vi "Graph Scale Properties.vi"(1 "Long term plot":refnum<vi>, 3 "Selected Variables":string[][](array[string]), 4 "Legend Rows":i32=5, 5 "error in (no error)":errorcluster, 6 "Short term graph":refnum<vi>) -> (19 "error out":errorcluster)   [LabVIEW 2013]
doc: "This vi sets the properties on event based (Scale range change, plot attributes change)\n[Input]\nlong term graph ref\nshort term graph ref\nselected variables array\nError in\n[output]\nError out"
panel:
  out "Array":u32[](array[colorbox])
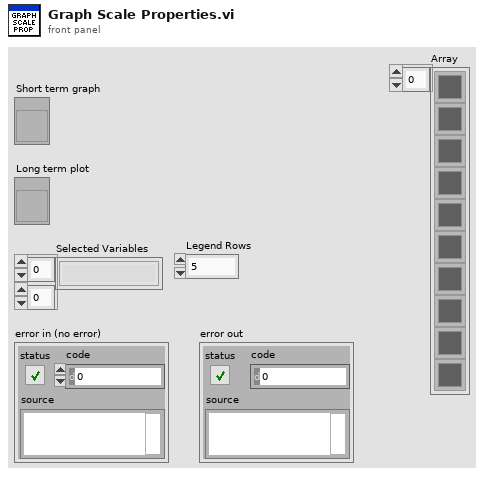
[diagram p1: front panel]
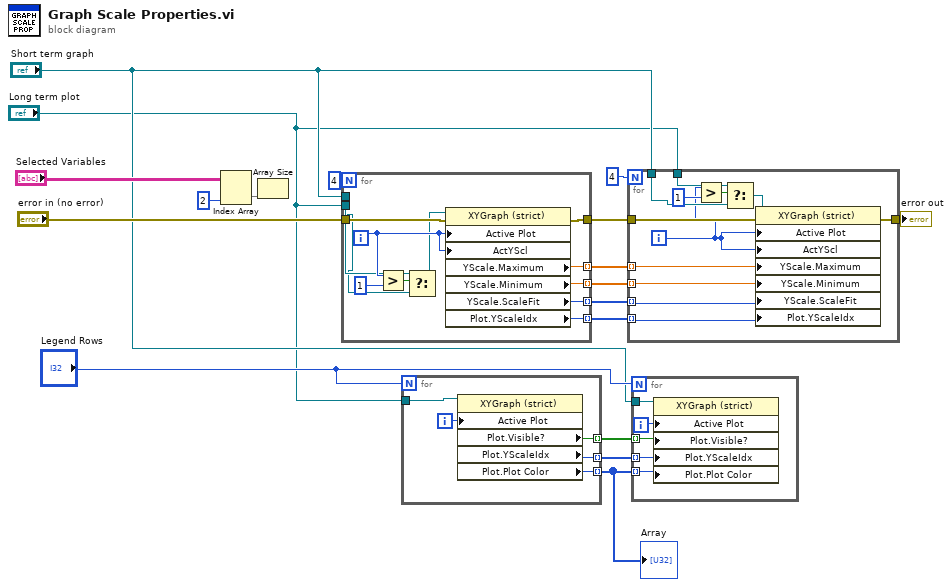
[diagram p0: block diagram]
diagram:
  n1 = Index Array(array="Selected Variables", index (col)=2 ("disabled index (col)")) -> (element=w12:string[])  [unwired: 1 in]
  n2 = Array Size(array=w12) -> ()  [unwired: 1 out]
  n3 = for {
    N: 4 -> [_]
    tunnel: "Long term plot" -> [w20]
    tunnel: "error in (no error)" -> [w30]
    tunnel: [w29] -> w13
    tunnel: [w28] -> w14 mode=indexing
    tunnel: [w27] -> w15 mode=indexing
    tunnel: [w26] -> w7 mode=indexing
    tunnel: [w25] -> w6 mode=indexing
    tunnel: "Short term graph" -> [w21]
    i -> [w23]
    n4 = Greater?(x=w23, y=1) -> (0:w22:bool)
    n5 = Select(t=w21, s=w22, f=w20) -> (s? t:f=w19:refnum<vi>)
    n6 = property class="XYGraph (strict)"(reference=w19, error in=w30, "Active Plot"=w23, "ActYScl"=w23) -> (error out=w29:errorcluster, "YScale.Maximum"=w28:dbl, "YScale.Minimum"=w27:dbl, "YScale.ScaleFit"=w26:u8, "Plot.YScaleIdx"=w25:u32)  [unwired: 1 out]
  }
  n7 = for {
    N: "Legend Rows" -> [_]
    tunnel: "Long term plot" -> [w35]
    tunnel: [w34] -> w18 mode=indexing
    tunnel: [w32] -> w5 mode=indexing
    tunnel: [w31] -> w3 mode=indexing
    i -> [w33]
    n8 = property class="XYGraph (strict)"(reference=w35, "Active Plot"=w33) -> ("Plot.Visible?"=w34:bool, "Plot.YScaleIdx"=w32:u32, "Plot.Plot Color"=w31:u32)  [unwired: 1 in, 2 out]
  }
  "Array" <- w3
  n9 = for {
    N: 4 -> [_]
    tunnel: "Short term graph" -> [w40]
    tunnel: w13 -> [w37]
    tunnel: [w47] -> w16
    tunnel: w14 -> [w46] mode=indexing
    tunnel: w15 -> [w45] mode=indexing
    tunnel: w7 -> [w44] mode=indexing
    tunnel: w6 -> [w43] mode=indexing
    tunnel: "Long term plot" -> [w39]
    i -> [w36]
    n10 = Greater?(x=w36, y=1) -> (0:w42:bool)
    n11 = Select(t=w39, s=w42, f=w40) -> (s? t:f=w38:refnum<vi>)
    n12 = property class="XYGraph (strict)"(reference=w38, error in=w37, "Active Plot"=w36, "ActYScl"=w36, "YScale.Maximum"=w46, "YScale.Minimum"=w45, "YScale.ScaleFit"=w44, "Plot.YScaleIdx"=w43) -> (error out=w47:errorcluster)  [unwired: 1 out]
  }
  "error out" <- w16
  n13 = for {
    N: "Legend Rows" -> [_]
    tunnel: "Short term graph" -> [w52]
    tunnel: w18 -> [w50] mode=indexing
    tunnel: w5 -> [w49] mode=indexing
    tunnel: w3 -> [w48] mode=indexing
    i -> [w51]
    n14 = property class="XYGraph (strict)"(reference=w52, "Active Plot"=w51, "Plot.Visible?"=w50, "Plot.YScaleIdx"=w49, "Plot.Plot Color"=w48) -> ()  [unwired: 1 in, 2 out]
  }
